vi "Get card Handle.vi"(4 "error in":errorcluster {"code" format="%.0x"}, 6 "板卡型号":string, 7 "Session":u32) -> (0 "error out":errorcluster, 2 "find？":bool, 3 "Output Handle":cluster{"Session":u32, "Card number":u32})   [LabVIEW 2018]
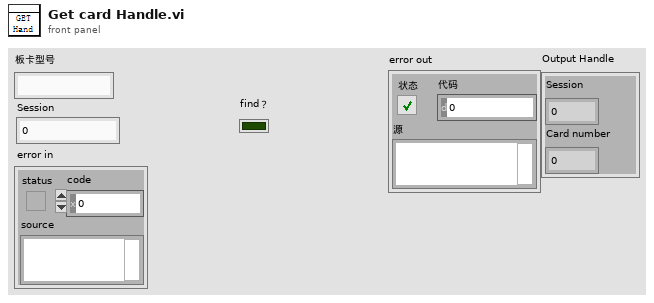
[diagram p1: front panel]
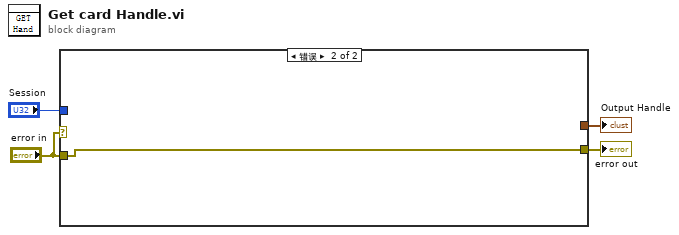
[diagram p0: block diagram]
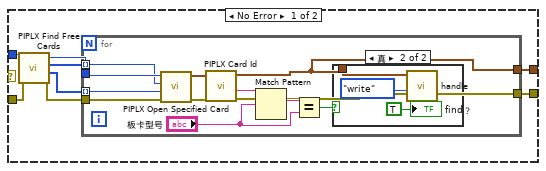
[diagram p2: hidden frame]
diagram:
  n1 = case shown="错误" "error in" {
    tunnel: "Session" -> [w8 _]
    tunnel: "error in" -> [w7 w28]
    tunnel: [w6 w28] -> w3
    tunnel: [w5 _] -> w1
    frame No Error {
      n2 = call <instrlib>:"PIPLX Find Free Cards.vi"("error in"=w7, "Session"=w8) -> ("error out"=w11:errorcluster, "Slot List"=w9:u32[], "Bus List"=w10:u32[], "Session out"=w12:u32)  [unwired: 6 in]
      n3 = for {
        tunnel: w12 -> [w24]
        tunnel: w11 -> [w21]
        tunnel: w10 -> [w16] mode=indexing
        tunnel: w9 -> [w15] mode=indexing
        tunnel: [w14] -> w5
        tunnel: [w13] -> w6
        n4 = call <instrlib>:"PIPLX Open Specified Card.vi"("error in"=w21, "Slot"=w15, "Bus"=w16, "Session"=w24) -> ("error out"=w23:errorcluster, "Output Handle"=w22:cluster{"Session":u32, "Card number":u32})  [unwired: 6 in]
        n5 = call <instrlib>:"PIPLX Card Id.vi"("error in"=w23, "Input Handle"=w22) -> ("error out"=w13:errorcluster, "Card ID"=w20:string, "Output Handle"=w14:cluster{"Session":u32, "Card number":u32})  [unwired: 7 in]
        n6 = Match Pattern(string=w20, regular expression="板卡型号") -> (match substring=w19:string)  [unwired: 1 in, 3 out]
        n7 = Equal?(x=w19, y="板卡型号") -> (x = y?=w17:bool)
        n8 = case shown="真" w17 {
          tunnel: w14 -> [_ w26]
          frame False {
          }
          frame True {
            n9 = call "handle.vi"("枚举"=enum16{"write", "read"}."write", "In Handle"=w26) -> ()  [unwired: 9 in, 1 out]
            "find？" <- TRUE ("find？")
          }
        }
      }
    }
    frame Error {
    }
  }
  "error out" <- w3
  "Output Handle" <- w1
